vi "get_tasks.vi"(8 "error in (no error)":errorcluster, 11 "DAQmxWriteSignals in":refnum<class "SignalWriterDL090202DAQmx.lvclass">) -> (0 "error out":errorcluster, 1 "counter tasks":refnum<k21>[](array[refnum]), 2 "output tasks":refnum<k21>[](array[refnum]), 3 "DAQmxWriteSignals out":refnum<class "SignalWriterDL090202DAQmx.lvclass">)   [LabVIEW 2010, in "SignalWriterDL090202DAQmx.lvclass"]
uses:
  SignalWriterDL090202DAQmx.lvclass
  class_data.vi
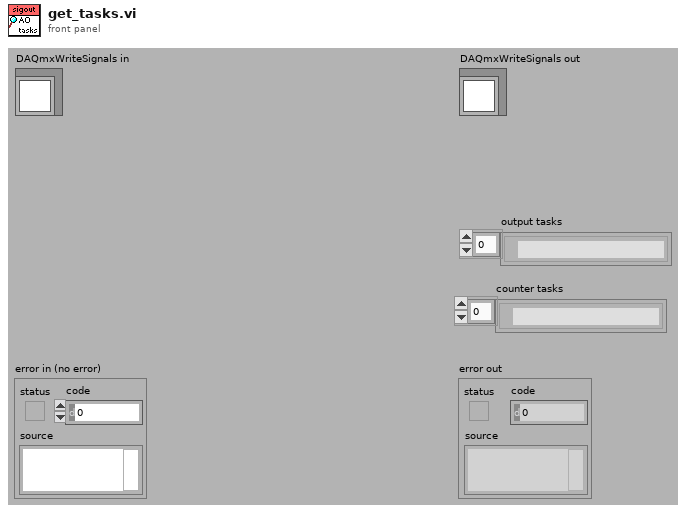
[diagram p1: front panel]
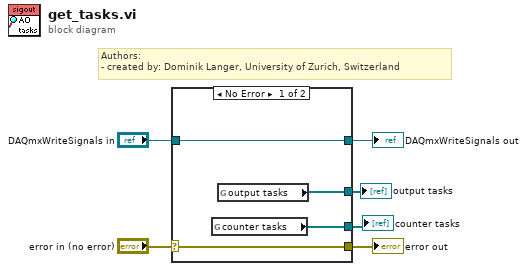
[diagram p0: block diagram]
diagram:
  # "Authors: \n- created by: Dominik Langer, University of Zurich, Switzerland"
  n1 = case shown="No Error" "error in (no error)" {
    selector: "error in (no error)" -> [w9 w12]
    tunnel: [w9 w12] -> w5
    tunnel: [w10 w11] -> w3
    tunnel: "DAQmxWriteSignals in" -> [w10 w11]
    tunnel: [w8 _] -> w2
    tunnel: [w7 _] -> w1
    frame No Error {
      n2 = global read "class_data.vi" "counter tasks"() -> (w7:refnum<k21>[])
      n3 = global read "class_data.vi" "output tasks"() -> (w8:refnum<k21>[])
    }
    frame Error {
    }
  }
  "error out" <- w5
  "DAQmxWriteSignals out" <- w3
  "output tasks" <- w2
  "counter tasks" <- w1
